vi "TDD - Get All Test Paths.vi"(8 "error in (no error)":errorcluster, 11 "Project in":refnum<vi>) -> (0 "error out":errorcluster, 2 "Test Paths":path[](array[path]))   [LabVIEW 2014]
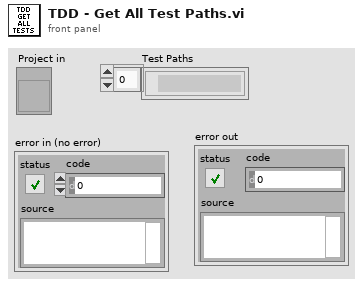
[diagram p1: front panel]
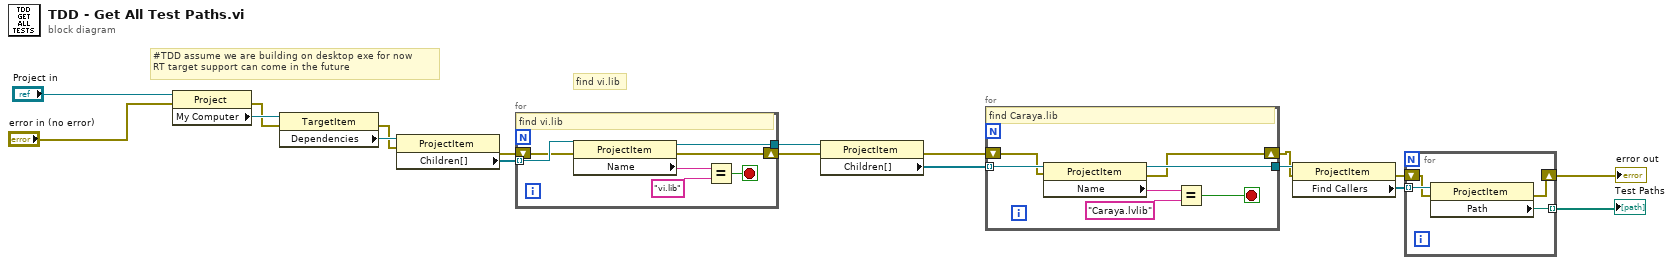
[diagram p0: block diagram]
diagram:
  # "find vi.lib"
  # "#TDD assume we are building on desktop exe for now\nRT target support can come in the future"
  n1 = property class="Project"(reference="Project in", error in="error in (no error)") -> (error out=w1:errorcluster, "My Computer"=w10:refnum<vi>)  [unwired: 1 out]
  n2 = property class="TargetItem"(reference=w10, error in=w1) -> (error out=w8:errorcluster, "Dependencies"=w11:refnum<vi>)  [unwired: 1 out]
  n3 = property class="ProjectItem"(reference=w11, error in=w8) -> (error out=w7:errorcluster, "Children[]"=w12:refnum<vi>[])  [unwired: 1 out]
  n4 = for {
    tunnel: w12 -> [w25] mode=indexing
    tunnel: [w21] -> w13
    shift-right: [w19] -> w6
    shift-left: w7 -> [w20]
    stop <- w22 stop-if-true
    # "find vi.lib"
    n5 = property class="ProjectItem"(reference=w25, error in=w20) -> (reference out=w21:refnum<vi>, error out=w19:errorcluster, "Name"=w24:string)
    n6 = Equal?(x=w24, y="vi.lib") -> (x = y?=w22:bool)
  }
  n7 = property class="ProjectItem"(reference=w13, error in=w6) -> (error out=w5:errorcluster, "Children[]"=w14:refnum<vi>[])  [unwired: 1 out]
  n8 = for {
    tunnel: w14 -> [w29] mode=indexing
    tunnel: [w28] -> w15
    shift-right: [w26] -> w4
    shift-left: w5 -> [w27]
    stop <- w30 stop-if-true
    # "find Caraya.lib"
    n9 = property class="ProjectItem"(reference=w29, error in=w27) -> (reference out=w28:refnum<vi>, error out=w26:errorcluster, "Name"=w32:string)
    n10 = Equal?(x=w32, y="Caraya.lvlib") -> (x = y?=w30:bool)
  }
  n11 = property class="ProjectItem"(reference=w15, error in=w4) -> (error out=w3:errorcluster, "Find Callers"=w16:refnum<vi>[])  [unwired: 1 out]
  n12 = for {
    tunnel: w16 -> [w36] mode=indexing
    tunnel: [w35] -> w17 mode=indexing
    shift-right: [w33] -> w2
    shift-left: w3 -> [w34]
    n13 = property class="ProjectItem"(reference=w36, error in=w34) -> (error out=w33:errorcluster, "Path"=w35:path)  [unwired: 1 out]
  }
  "Test Paths" <- w17
  "error out" <- w2
